vi "CMN Cal.vi"(8 "error in (no error)":errorcluster, 10 "TC Type":T1(ring)=enum."CF_Z_Bridge") -> (0 "error out":errorcluster, 2 "C0, C1":dbl[](array[numeric]))   [LabVIEW 2016]
uses:
  <vilib>/Utility/file.llb/Write Delimited Spreadsheet (DBL).vi
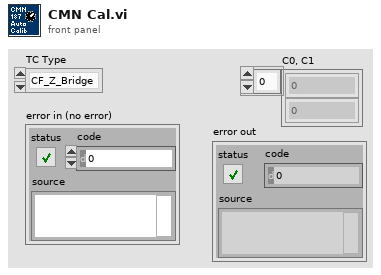
[diagram p1: front panel]
types:
  T1 = enum16{"CF", "CF_Z_Bridge", "MNK", "MNK_Z_Bridge"}
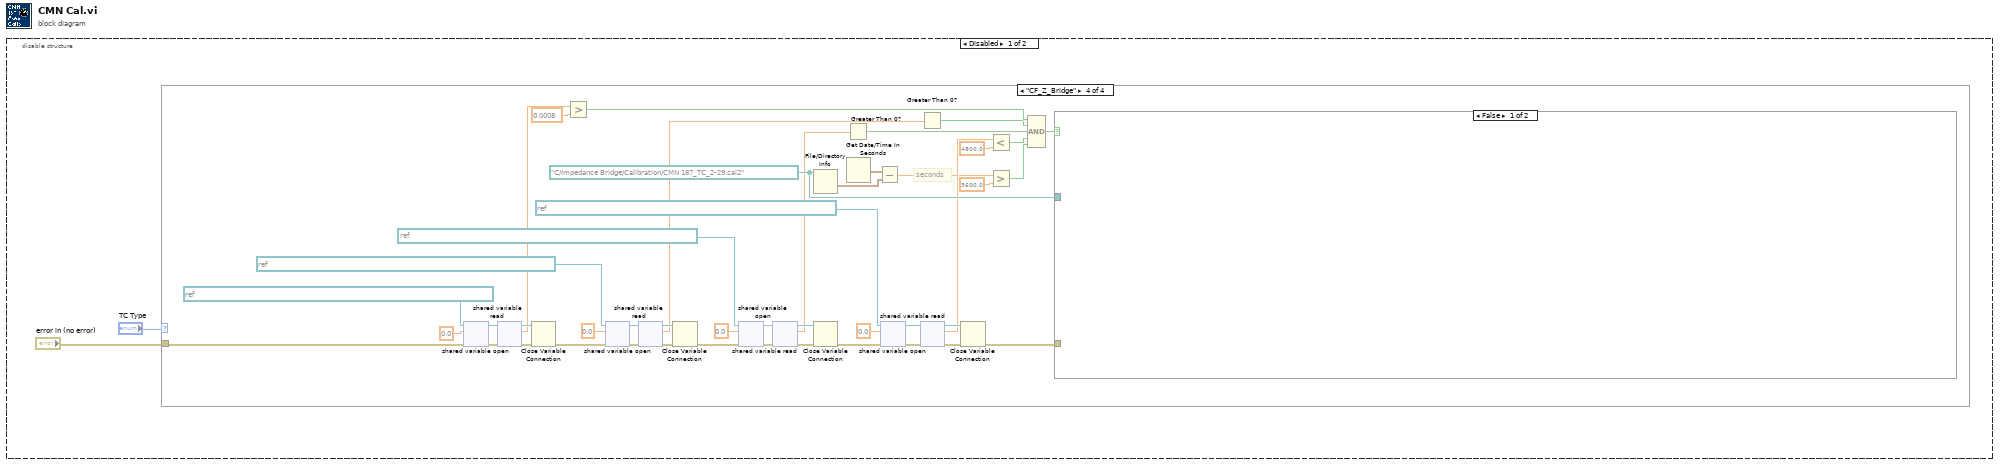
[diagram p0: block diagram]
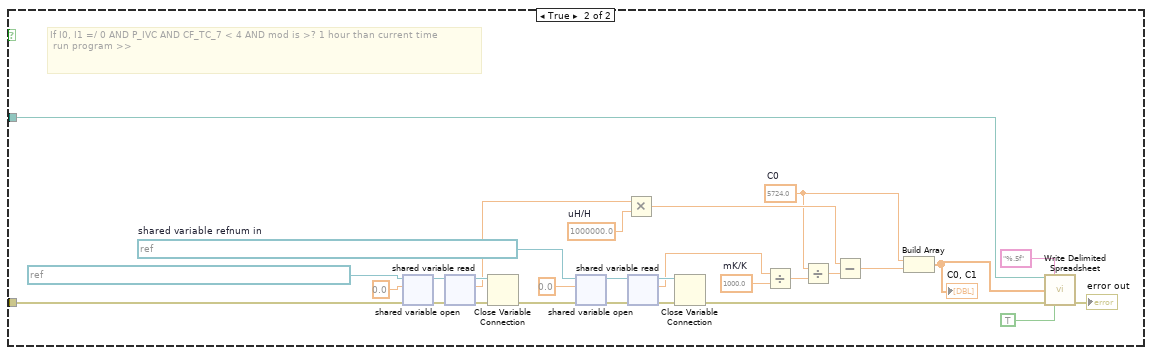
[diagram p5: hidden frame]
diagram:
  n1 = disable-structure shown="Disabled" {
    frame Disabled {
      n2 = case shown="\"CF_Z_Bridge\"" "TC Type" {
        tunnel: "error in (no error)" -> [_ _ _ w9]
        frame "CF", Default {
        }
        frame "MNK" {
        }
        frame "MNK_Z_Bridge" {
        }
        frame "CF_Z_Bridge" {
          w48 = path "C:/Impedance Bridge/Calibration/CMN 187_TC_2-29.cal2" ("file path (dialog if empty)")
          # "seconds"
          n3 = shared-variable-open(refnum<k21> "ni.var.psp://housesoftheholy/Leiden CF900/Leiden CF FP/CF FP MG3" ("shared variable refnum in"), w9, 0.0 ("y")) -> (w35:refnum<k21>, w33:errorcluster)  [unwired: 1 in]
          n4 = shared-variable-read(w35, w33) -> (w34:refnum<k21>, w32:errorcluster, w29:dbl)  [unwired: 1 out]
          n5 = Close Variable Connection(8:w32, 11:w34) -> (0:w8:errorcluster)
          n6 = Greater?(x=w29, y=0.0008) -> (0:w27:bool)
          n7 = shared-variable-open(refnum<k21> "ni.var.psp://housesoftheholy/Leiden CF900/Leiden CF TC/CF TC I0" ("shared variable refnum in"), w8, 0.0 ("y")) -> (w47:refnum<k21>, w45:errorcluster)  [unwired: 1 in]
          n8 = shared-variable-read(w47, w45) -> (w46:refnum<k21>, w44:errorcluster, w4:dbl)  [unwired: 1 out]
          n9 = Close Variable Connection(8:w44, 11:w46) -> (0:w7:errorcluster)
          n10 = shared-variable-open(refnum<k21> "ni.var.psp://housesoftheholy/Leiden CF900/Leiden CF TC/CF TC I1" ("shared variable refnum in"), w7, 0.0 ("y")) -> (w41:refnum<k21>, w39:errorcluster)  [unwired: 1 in]
          n11 = shared-variable-read(w41, w39) -> (w40:refnum<k21>, w38:errorcluster, w3:dbl)  [unwired: 1 out]
          n12 = File/Directory Info(path=w48) -> (last mod=w14:timestamp)  [unwired: 1 in, 6 out]
          n13 = Close Variable Connection(8:w38, 11:w40) -> (0:w6:errorcluster)
          n14 = Greater Than 0?(x=w3) -> (x > 0?=w25:bool)
          n15 = Get Date/Time In Seconds() -> (seconds since 1Jan1904=w15:timestamp)
          n16 = Subtract(x=w15, y=w14) -> (x-y=w13:dbl)
          n17 = shared-variable-open(refnum<k21> "ni.var.psp://housesoftheholy/Leiden CF900/Leiden CF TC/CF TC T7" ("shared variable refnum in"), w6, 0.0 ("y")) -> (w18:refnum<k21>, w20:errorcluster)  [unwired: 1 in]
          n18 = Greater Than 0?(x=w4) -> (x > 0?=w26:bool)
          n19 = shared-variable-read(w18, w20) -> (w19:refnum<k21>, w21:errorcluster, w17:dbl)  [unwired: 1 out]
          n20 = Close Variable Connection(8:w21, 11:w19) -> (0:w5:errorcluster)
          n21 = Less?(x=w17, y=4800.0) -> (x < y?=w10:bool)
          n22 = Greater?(x=w13, y=3600.0) -> (0:w11:bool)
          n23 = Compound Arithmetic op=AND(w27, w26, w25, w10, w11) -> (w24:bool)
          n24 = case shown="False" w24 {
            tunnel: w48 -> [_ w57]
            tunnel: w5 -> [_ w53]
            frame False {
            }
            frame True {
              w55 = 1000.0  # mK/K
              w62 = refnum<k21> "ni.var.psp://housesoftheholy/Leiden CF900/Leiden CF TC/CF TC T7"  # shared variable refnum in
              w76 = 1000000.0  # uH/H
              w74 = 5724.0  # C0
              # "If I0, I1 =/ 0 AND P_IVC AND CF_TC_7 < 4 AND mod is >? 1 hour than current time\n run program >>"
              n25 = shared-variable-open(refnum<k21> "ni.var.psp://housesoftheholy/Leiden CF900/CF_TC_Z_R0" ("shared variable refnum in"), w53, 0.0 ("y")) -> (w69:refnum<k21>, w67:errorcluster)  [unwired: 1 in]
              n26 = shared-variable-read(w69, w67) -> (w68:refnum<k21>, w66:errorcluster, w64:dbl)  [unwired: 1 out]
              n27 = Close Variable Connection(8:w66, 11:w68) -> (0:w52:errorcluster)
              n28 = shared-variable-open(w62, w52, 0.0 ("y")) -> (w58:refnum<k21>, w60:errorcluster)  [unwired: 1 in]
              n29 = Multiply(x=w64, y=w76) -> (x*y=w75:dbl)
              n30 = shared-variable-read(w58, w60) -> (w59:refnum<k21>, w61:errorcluster, w56:dbl)  [unwired: 1 out]
              n31 = Close Variable Connection(8:w61, 11:w59) -> (0:w51:errorcluster)
              n32 = Divide(x=w56, y=w55) -> (x/y=w54:dbl)
              n33 = Divide(x=w74, y=w54) -> (x/y=w77:dbl)
              n34 = Subtract(x=w75, y=w77) -> (x-y=w73:dbl)
              n35 = Build Array(w74, w73) -> (w72:dbl[])
              "C0, C1" <- w72
              n36 = call-poly <vilib>:"Write Delimited Spreadsheet.vi"("file path (dialog if empty)"=w57, "format (%.3f)"="%.5f", "1D data"=w72, "error in (no error)"=w51, "transpose? (no:F)"=TRUE) -> ("error out"=→"error out":errorcluster)  [unwired: 9 in, 1 out]
            }
          }
        }
      }
    }
    frame Enabled {
    }
  }
